vi "start list.vi"(8 "error in (no error)":errorcluster, 10 "time":dbl, 11 "identifier":string) -> (0 "error out":errorcluster, 3 "function return":u32)   [LabVIEW 2015, in "XGL_DPP.lvlib"]
doc: "EXTERN DECLSPEC uint32_t CALL_CONV start_list(const char * identifier, const double time);"
uses:
  XGL_DPP.lvlib
  XGL_DPP.dll
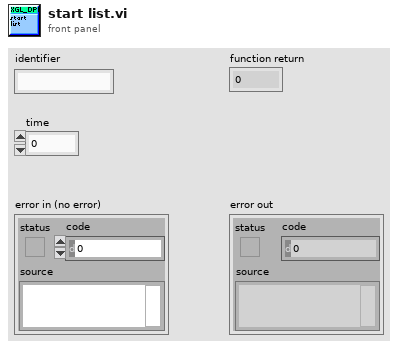
[diagram p1: front panel]
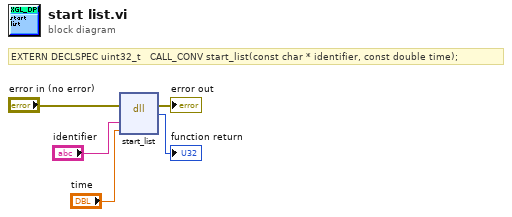
[diagram p0: block diagram]
diagram:
  # "EXTERN DECLSPEC uint32_t   CALL_CONV start_list(const char * identifier, const double time);"
  n1 = dll-call lib="D:/Users/XRF/Desktop/Scanning Software_Demokritos_2015_v7/libs/Vis_2/XGL_DPP.*" fn="start_list"(error in="error in (no error)", "identifier"="identifier", "time"="time") -> (error out=→"error out":errorcluster, →"function return":u32)  [unwired: 4 in, 1 out]
